vi "Priority Index.vi"(11 "MB status":T1[](array[typedef]) {"MB update(s)" format="%.2g"; "ProCoDA Request"."PC update (s)" format="%.2f"; "ProCoDA Request"."# registers" min=1}) -> (0 "Priority Index":i32, 1 "wait (ms)":i32)   [LabVIEW 2019]
uses:
  MB status.ctl
  ProCoDA MB Request.ctl
  Read Write.ctl
panel:
  out "Delay (s)":dbl[](array[numeric])
  out "Next updates (s)":dbl[](array[numeric])
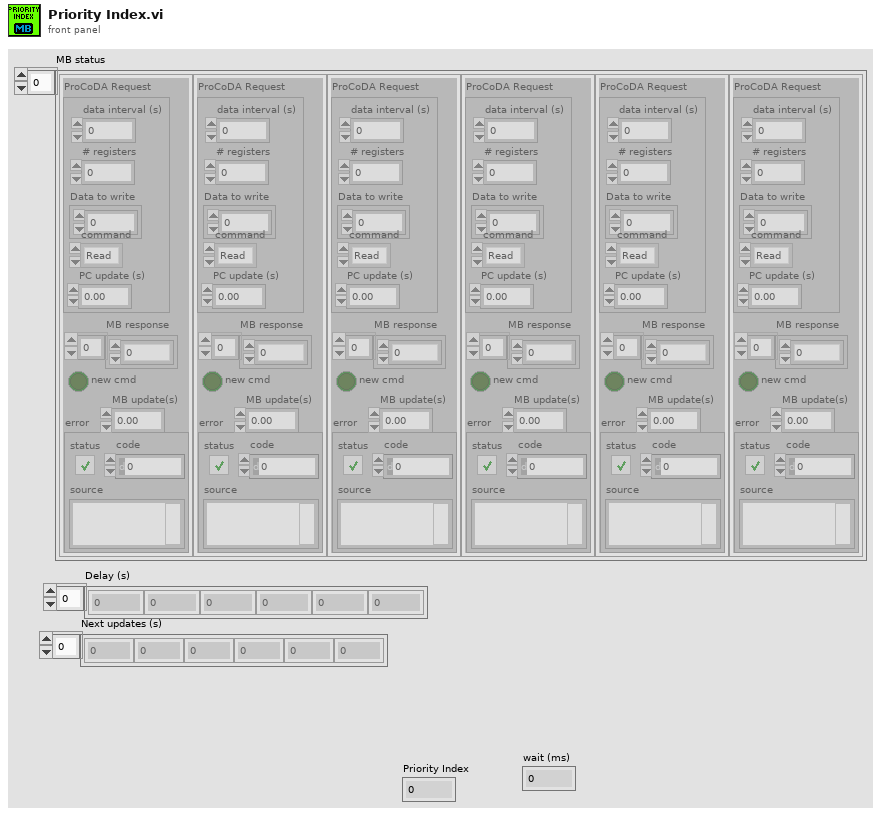
[diagram p1: front panel]
types:
  T1 = typedef "MB status.ctl" = cluster{"ProCoDA Request":T2, "MB response":dbl[], "new cmd":bool, "error":errorcluster, "MB update(s)":dbl}
  T2 = typedef "ProCoDA MB Request.ctl" = cluster{"# registers":u8, "Data to write":u16[], "data interval (s)":dbl, "command":T3, "PC update (s)":dbl}
  T3 = typedef "Read Write.ctl" = enum16{"Read", "Write"}
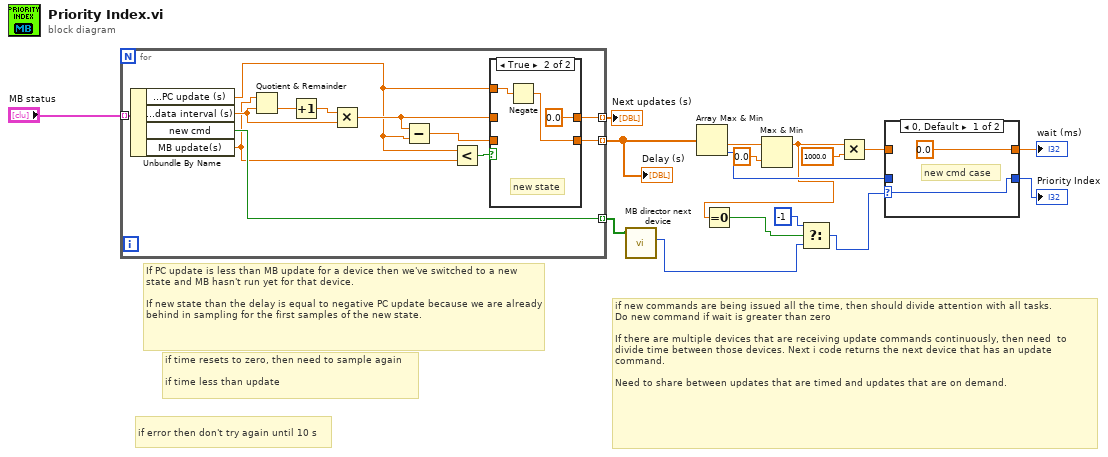
[diagram p0: block diagram]
diagram:
  # "if error then don't try again until 10 s"
  # "If PC update is less than MB update for a device then we've switched to a new state and MB hasn't run yet for that device.\n\nIf new state than the delay is equal to negative PC update because we are already behind in sampling for the first samples of the new state."
  # "if new commands are being issued all the time, then should divide attention with all tasks.\nDo new command if wait is greater than zero\n\nIf there are multiple devices that are receiving update commands continuously, then need  to divide time between those devices. Next i code returns the next device that has an update command.\n\nNeed to share between updates that are timed and updates that are on demand."
  # "if time resets to zero, then need to sample again\n\nif time less than update"
  n1 = for {
    tunnel: [w26] -> w5 mode=indexing
    tunnel: [w25] -> w15 mode=indexing
    tunnel: "MB status" -> [w23] mode=indexing
    tunnel: [w21] -> w11 mode=indexing
    n2 = Unbundle By Name(w23) -> ("ProCoDA Request.PC update (s)"=w17:dbl, "ProCoDA Request.data interval (s)"=w24:dbl, "new cmd"=w21:bool, "MB update(s)"=w19:dbl)
    n3 = Quotient & Remainder(x=w19, y=w24) -> (floor(x/y)=w22:dbl)  [unwired: 1 out]
    n4 = Increment(x=w22) -> (x+1=w28:dbl)
    n5 = Multiply(x=w28, y=w24) -> (x*y=w18:dbl)
    n6 = Subtract(x=w18, y=w17) -> (x-y=w20:dbl)
    n7 = Less?(x=w17, y=w19) -> (x < y?=w27:bool)
    n8 = case shown="True" w27 {
      tunnel: w20 -> [w30 _]
      tunnel: [w30 w31] -> w26
      tunnel: w18 -> [w29 _]
      tunnel: [w29 0.0] -> w25
      tunnel: w17 -> [_ w32]
      frame False {
      }
      frame True {
        # "new state"
        n9 = Negate(x=w32) -> (-x=w31:dbl)
      }
    }
  }
  "Next updates (s)" <- w15
  "Delay (s)" <- w5
  n10 = call "MB director next device.vi"("New cmd"=w11) -> ("Next priority index"=w2:i32)  [unwired: 5 in, 1 out]
  n11 = Array Max & Min(array=w5) -> (min value=w12:dbl, min index (indices)=w6:i32)  [unwired: 2 out]
  n12 = Max & Min(x=w12, y=0.0) -> (max(x,y)=w4:dbl)  [unwired: 1 out]
  n13 = Equal To 0?(x=w4) -> (x = 0?=w1:bool)
  n14 = Select(t=-1, s=w1, f=w2) -> (s? t:f=w10:i32)
  n15 = Multiply(x=w4, y=1000.0) -> (x*y=w7:dbl)
  n16 = case shown="0, Default" w10 {
    selector: w10 -> [w35 _]
    tunnel: [w35 w37] -> w9
    tunnel: w6 -> [_ w37]
    tunnel: [0.0 w36] -> w8
    tunnel: w7 -> [_ w36]
    frame 0, Default {
      # "new cmd case"
    }
    frame -1 {
    }
  }
  "wait (ms)" <- w8
  "Priority Index" <- w9
